vi "Test ConfigurableQMH API.vi"() -> ()   [LabVIEW 2014]
doc: "ConfigurableQMH API Tester."
uses:
  ModuleConfiguration--Cluster.ctl
  ConfigurableQMH.lvlib
panel:
  in  "Active Modules":i32(listbox)
  in  "New Module Name":string
  in  "Modify Configuration":bool
  in  "Configuration":T1
  in  "Run as Singleton?":bool
  in  "Show Block Diagram":bool
  in  "Refresh Modules":bool
  in  "Stop Module":bool
  in  "Run New Module":bool
  in  "Hide Module Panel":bool
  in  "Show Module Panel":bool
  out "Status":string
  # "This VI tests the API for the Module."
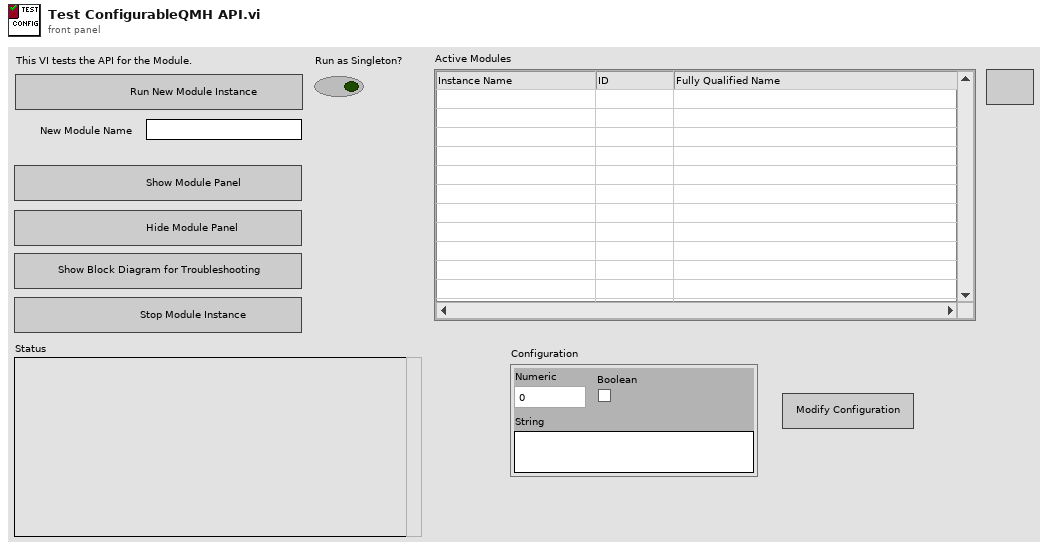
[diagram p1: front panel]
types:
  T1 = typedef "ConfigurableQMH.lvlib/ModuleConfiguration--Cluster.ctl" = cluster{"Numeric":dbl, "Boolean":bool, "String":string}
  T2 = typedef "ConfigurableQMH.lvlib/Broadcast Events--cluster.ctl" = cluster{"Module Did Init":refnum<user-event>, "Status Updated":refnum<user-event>, "Error Reported":refnum<user-event>, "Module Did Stop":refnum<user-event>, "Update Module Execution Status":refnum<user-event>, "Module Configuration":refnum<user-event>}
  T3 = typedef "ConfigurableQMH.lvlib/GetConfiguration (Reply Payload)--cluster.ctl" = cluster{"Configuration":T1, "GetConfiguration_error":errorcluster}
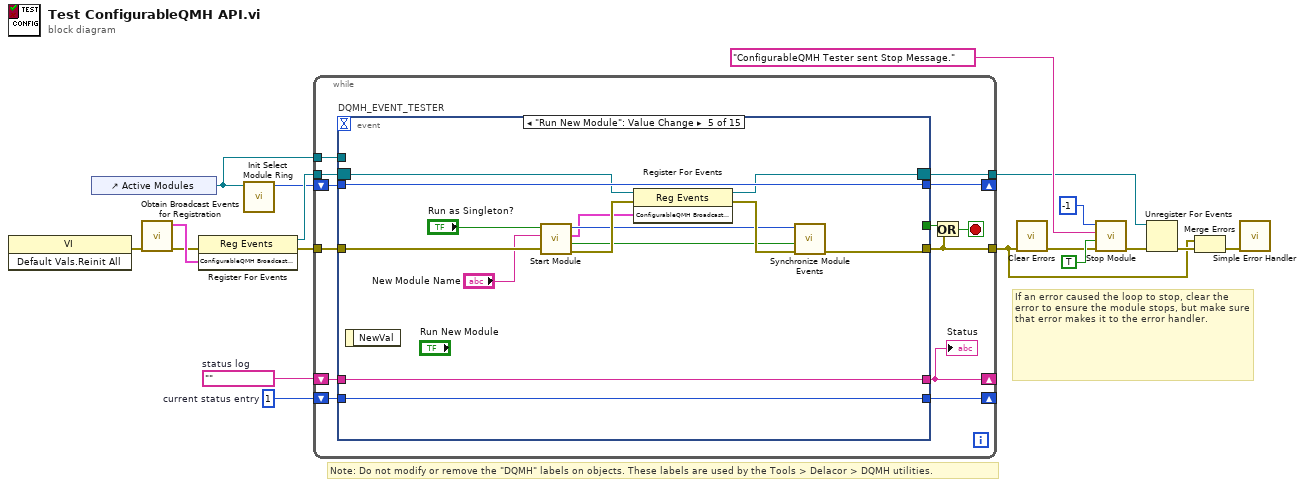
[diagram p0: block diagram]
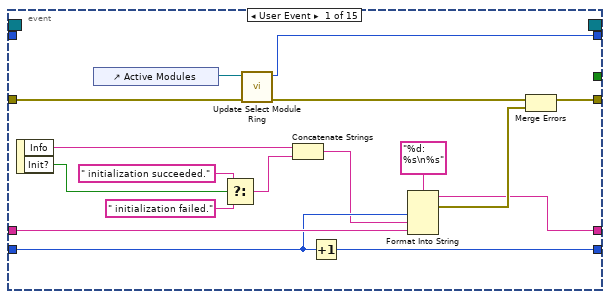
[diagram p2: hidden frame]
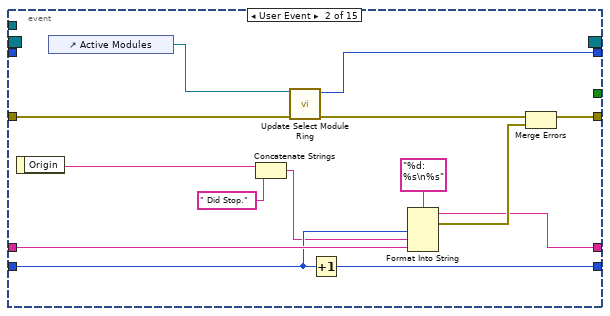
[diagram p3: hidden frame]
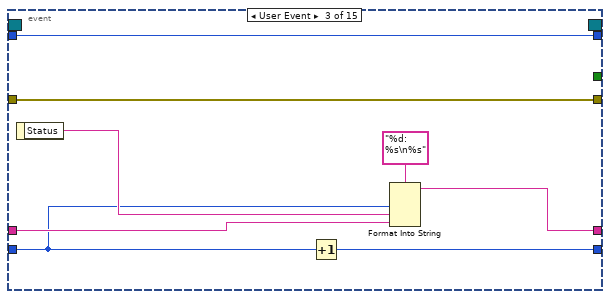
[diagram p4: hidden frame]
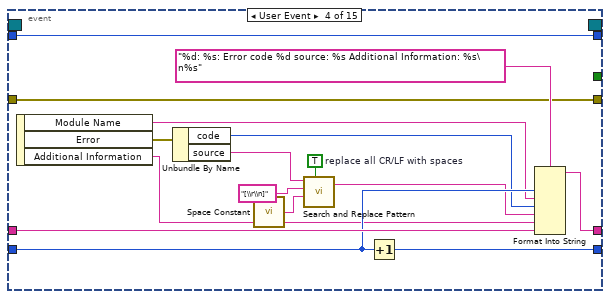
[diagram p5: hidden frame]
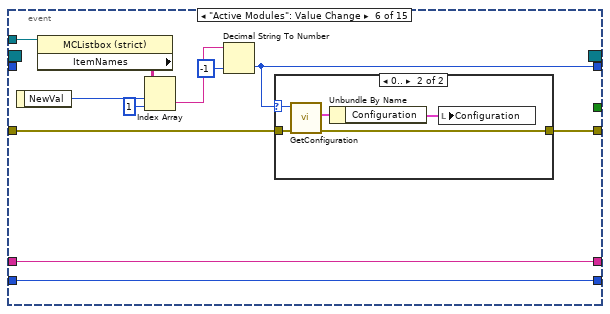
[diagram p6: hidden frame]
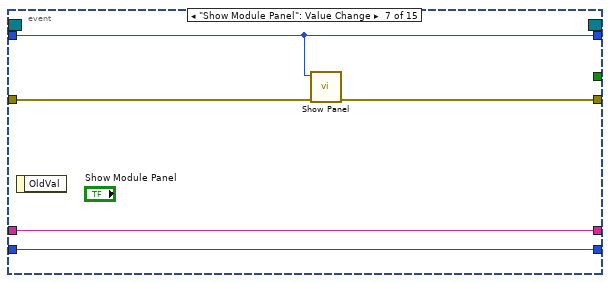
[diagram p8: hidden frame]
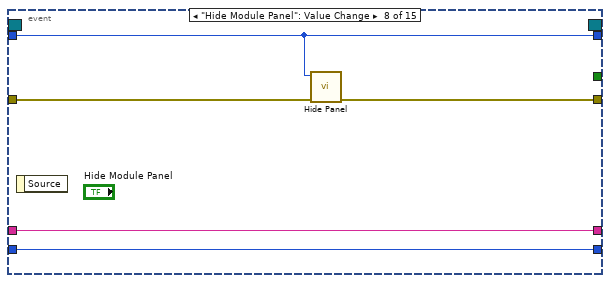
[diagram p9: hidden frame]
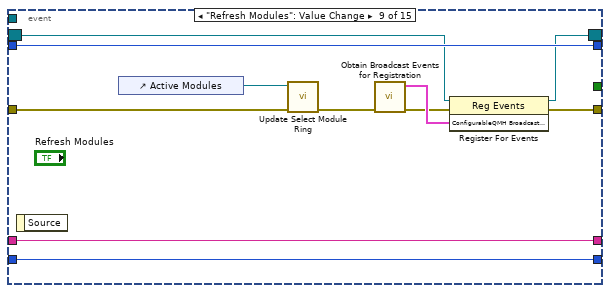
[diagram p10: hidden frame]
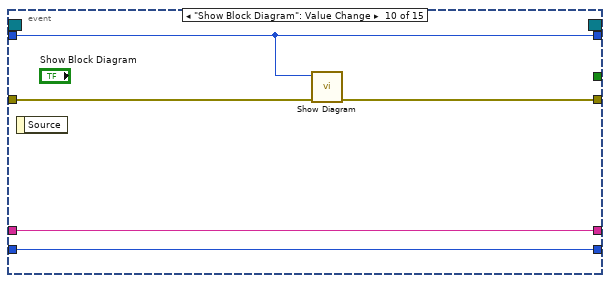
[diagram p11: hidden frame]
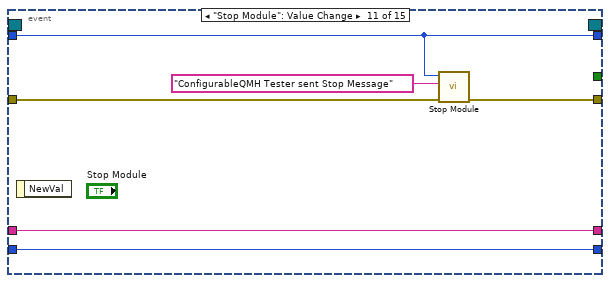
[diagram p12: hidden frame]
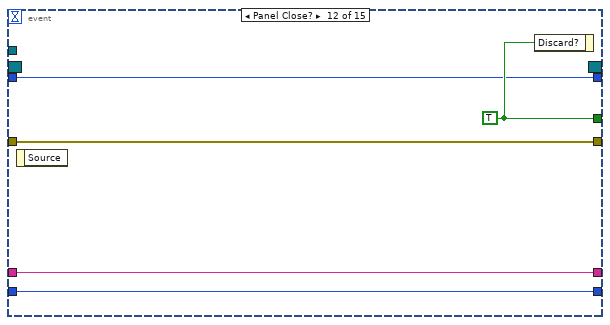
[diagram p13: hidden frame]
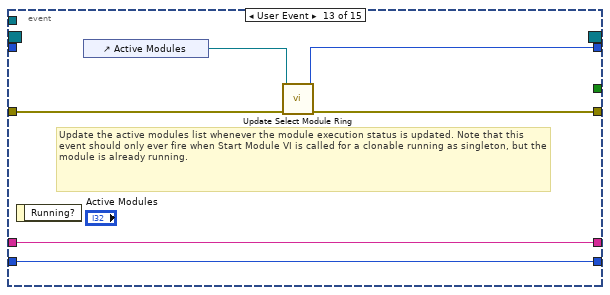
[diagram p14: hidden frame]
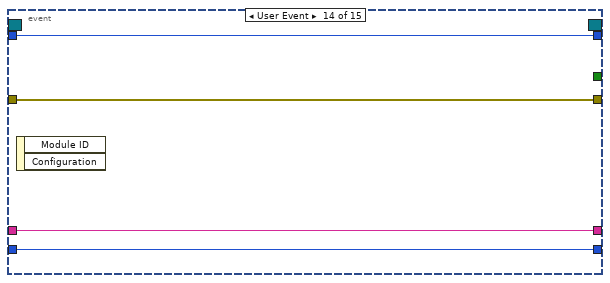
[diagram p15: hidden frame]
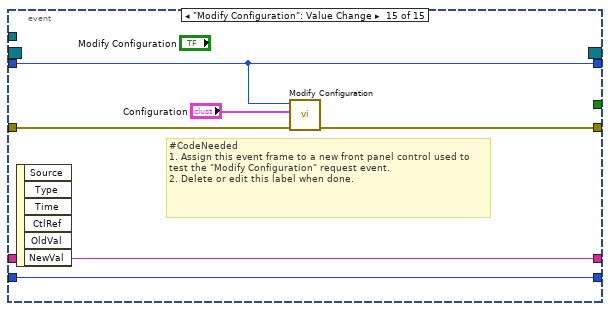
[diagram p16: hidden frame]
diagram:
  w14 = 1  # current status entry
  w15 = ""  # status log
  # "If an error caused the loop to stop, clear the error to ensure the module stops, but make sure that error makes it to the error handler."
  # "Note: Do not modify or remove the \"DQMH\" labels on objects. These labels are used by the Tools > Delacor > DQMH utilities."
  n1 = invoke class="VI" method="Default Vals.Reinit All"() -> (error out=w3:errorcluster)  [unwired: 3 in, 2 out]
  n2 = control-ref of="Active Modules"() -> (w1:refnum<vi>)
  n3 = call "Obtain Broadcast Events for Registration.vi"("error in (no error)"=w3) -> ("error out"=w2:errorcluster, "ConfigurableQMH Broadcast Events"=w12:T2)  [unwired: 9 in]
  n4 = register-events(error in=w2, w12) -> (reference out=w18:refnum<event-registration>, error out=w11:errorcluster)  [unwired: 1 in]
  n5 = call "Init Select Module Ring.vi"("Select Module MCL Ref"=w1) -> ("Value for All Modules"=w13:i32)  [unwired: 8 in, 2 out]
  n6 = while {
    tunnel: w18 -> [w31]
    tunnel: [w20] -> w4
    tunnel: w11 -> [w29]
    shift-right: [w25] -> _
    shift-left: w15 -> [w27]
    shift-right: [w26] -> _
    shift-left: w14 -> [w28]
    shift-right: [w22] -> _
    shift-left: w13 -> [w23]
    tunnel: [w21] -> w8
    tunnel: w1 -> [w19]
    stop <- w24 stop-if-true
    n7 = event "DQMH_EVENT_TESTER" shown="[4] \"Run New Module\": Value Change" {
      selector: w31 -> [_ _ _ _ w94 _ _ _ w134 _ _ _ _ _ _]
      dyn-events: [_ _ _ _ w93 _ _ _ w133 _ _ _ _ _ _] -> w21
      timeout: _ -> [_ _ _ _ _ _ _ _ _ _ _ _ _ _ _]
      tunnel: [_ _ _ _ _ _ _ _ _ _ _ w154 _ _ _] -> w30
      tunnel: [w39 w54 w70 w76 w92 w102 w121 w126 w128 w140 w145 w153 w157 w164 w167] -> w20
      tunnel: w29 -> [w40 w56 w70 w76 w95 w103 w122 w127 w135 w143 w146 w153 w158 w164 w170]
      tunnel: w28 -> [w45 w59 w63 w82 w97 w110 w119 w124 w137 w141 w148 w151 w159 w162 w168]
      tunnel: w27 -> [w46 w60 w66 w84 w98 w111 w120 w125 w138 w142 w149 w152 w160 w163 w169]
      tunnel: [w43 w57 w67 w79 w98 w111 w120 w125 w138 w142 w149 w152 w160 w163 w169] -> w25
      tunnel: [w44 w58 w69 w85 w97 w110 w119 w124 w137 w141 w148 w151 w159 w162 w168] -> w26
      tunnel: w23 -> [_ _ w64 w86 w96 _ w118 w123 w136 w139 w147 w150 _ w161 w166]
      tunnel: [w38 w53 w64 w86 w96 w101 w118 w123 w136 w139 w147 w150 w155 w161 w166] -> w22
      tunnel: w19 -> [_ _ _ _ _ w104 _ _ _ _ _ _ _ _ _]
      event User Event {
        n8 = event-data() -> ("Info"=w42:string, "Init?"=w35:bool)  [unwired: 1 in]
        n9 = control-ref of="Active Modules"() -> (w32:refnum<vi>)
        n10 = Select(t=" initialization succeeded.", s=w35, f=" initialization failed.") -> (s? t:f=w34:string)
        n11 = call "Update Select Module Ring.vi"("error in (no error)"=w40, "Select Module MCL Ref"=w32) -> ("error out"=w33:errorcluster, "New Module Ring Value"=w38:i32)  [unwired: 8 in]
        n12 = Concatenate Strings(w42, w34) -> (w41:string)
        n13 = Increment(x=w45) -> (x+1=w44:i32)
        n14 = Format Into String(format string="%d: %s\n%s", w45, w41, w46) -> (resulting string=w43:string, error out=w48:errorcluster)  [unwired: 2 in]
        n15 = Merge Errors(w33, w48) -> (w39:errorcluster)
      }
      event User Event {
        n16 = event-data() -> ("Origin"=w51:string)  [unwired: 1 in]
        n17 = control-ref of="Active Modules"() -> (w49:refnum<vi>)
        n18 = Concatenate Strings(w51, " Did Stop.") -> (w50:string)
        n19 = call "Update Select Module Ring.vi"("error in (no error)"=w56, "Select Module MCL Ref"=w49) -> ("error out"=w55:errorcluster, "New Module Ring Value"=w53:i32)  [unwired: 8 in]
        n20 = Increment(x=w59) -> (x+1=w58:i32)
        n21 = Format Into String(format string="%d: %s\n%s", w59, w50, w60) -> (resulting string=w57:string, error out=w62:errorcluster)  [unwired: 2 in]
        n22 = Merge Errors(w55, w62) -> (w54:errorcluster)
      }
      event User Event {
        n23 = event-data() -> ("Status"=w65:string)  [unwired: 1 in]
        n24 = Increment(x=w63) -> (x+1=w69:i32)
        n25 = Format Into String(format string="%d: %s\n%s", w63, w65, w66) -> (resulting string=w67:string)  [unwired: 2 in, 1 out]
      }
      event User Event {
        w80 = TRUE  # replace all CR/LF with spaces
        n26 = event-data() -> ("Module Name"=w74:string, "Error"=w73:errorcluster, "Additional Information"=w71:string)  [unwired: 1 in]
        n27 = Unbundle By Name(w73) -> ("code"=w75:i32, "source"=w77:string)
        n28 = call <vilib>:"Space Constant.vi"() -> ("String"=w81:string)
        n29 = call <vilib>:"Search and Replace Pattern.vi"("string"=w77, "regular expression (\"\")"="[\\r\\n]" ("regular expression (\"\")"), "replace string (\"\")"=w81, "replace all? (F)"=w80) -> ("result string"=w78:string)  [unwired: 1 in, 1 out]
        n30 = Increment(x=w82) -> (x+1=w85:i32)
        n31 = Format Into String(format string="%d: %s: Error code %d source: %s Additional Information: %s\n%s", w82, w74, w75, w78, w71, w84) -> (resulting string=w79:string)  [unwired: 2 in, 1 out]
      }
      event "Run New Module": Value Change {
        n32 = event-data() -> ()  [unwired: 1 in, 1 out]
        n33 = call "Start Module.vi"("error in (no error)"=w95, "Module Name (empty: default)"="New Module Name", "Run as Singleton? (F)"="Run as Singleton?") -> ("error out"=w99:errorcluster, "Wait for Event Sync?"=w90:bool, "ConfigurableQMH Broadcast Events"=w89:T2, "Module ID"=w91:i32)  [unwired: 5 in]
        n34 = register-events(reference=w94, error in=w99, w89) -> (reference out=w93:refnum<event-registration>, error out=w100:errorcluster)
        n35 = call "Synchronize Module Events.vi"("error in (no error)"=w100, "Wait for Event Sync?"=w90, "Module ID"=w91) -> ("error out"=w92:errorcluster)  [unwired: 7 in, 1 out]
      }
      event "Active Modules": Value Change {
        n36 = event-data() -> ("NewVal"=w108:i32)  [unwired: 1 in]
        n37 = property class="MCListbox (strict)"(reference=w104) -> ("ItemNames"=w109:string[][])  [unwired: 1 in, 2 out]
        n38 = Index Array(array=w109, index (row)=w108, index (col)=1 ("disabled index (col)")) -> (element=w106:string)
        n39 = Decimal String To Number(string=w106, default (0L)=-1 ("default (0 I32)")) -> (number=w101:i32)  [unwired: 1 in, 1 out]
        n40 = case shown="0.." w101 {
          selector: w101 -> [_ w113]
          tunnel: w103 -> [w112 w115]
          tunnel: [w112 w114] -> w102
          frame Default {
          }
          frame 0.. {
            n41 = call "GetConfiguration.vi"("error in (no error)"=w115, "Module ID"=w113) -> ("error out"=w114:errorcluster, "Reply Payload"=w117:T3)  [unwired: 7 in, 1 out]
            n42 = Unbundle By Name(w117) -> ("Configuration"=w116:T1)
            n43 = local write "Configuration"(w116) -> ()
          }
        }
      }
      event "Show Module Panel": Value Change {
        n44 = event-data() -> ()  [unwired: 1 in, 1 out]
        n45 = call "Show Panel.vi"("error in (no error)"=w122, "Module ID"=w118) -> ("error out"=w121:errorcluster)  [unwired: 9 in]
      }
      event "Hide Module Panel": Value Change {
        n46 = event-data() -> ()  [unwired: 1 in, 1 out]
        n47 = call "Hide Panel.vi"("error in (no error)"=w127, "Module ID"=w123) -> ("error out"=w126:errorcluster)  [unwired: 9 in]
      }
      event "Refresh Modules": Value Change {
        n48 = event-data() -> ()  [unwired: 1 in, 1 out]
        n49 = control-ref of="Active Modules"() -> (w130:refnum<vi>)
        n50 = call "Update Select Module Ring.vi"("error in (no error)"=w135, "Select Module MCL Ref"=w130) -> ("error out"=w131:errorcluster)  [unwired: 8 in, 1 out]
        n51 = call "Obtain Broadcast Events for Registration.vi"("error in (no error)"=w131) -> ("error out"=w129:errorcluster, "ConfigurableQMH Broadcast Events"=w132:T2)  [unwired: 9 in]
        n52 = register-events(reference=w134, error in=w129, w132) -> (reference out=w133:refnum<event-registration>, error out=w128:errorcluster)
      }
      event "Show Block Diagram": Value Change {
        n53 = event-data() -> ()  [unwired: 1 in, 1 out]
        n54 = call "Show Diagram.vi"("error in (no error)"=w143, "Module ID"=w139) -> ("error out"=w140:errorcluster)  [unwired: 9 in]
      }
      event "Stop Module": Value Change {
        n55 = event-data() -> ()  [unwired: 1 in, 1 out]
        n56 = call "Stop Module.vi"("error in (no error)"=w146, "Origin"="ConfigurableQMH Tester sent Stop Message", "Module ID"=w147) -> ("error out"=w145:errorcluster)  [unwired: 8 in]
      }
      event Panel Close? {
        w154 = TRUE ("Discard?")
        n57 = event-data() -> ()  [unwired: 1 in, 1 out]
        n58 = event-data("Discard?"=w154) -> ()  [unwired: 1 in, 1 out]
      }
      event User Event {
        # "Update the active modules list whenever the module execution status is updated. Note that this event should only ever fire when Start Module VI is called for a clonable running as singleton, but the module is already running."
        n59 = event-data() -> ()  [unwired: 1 in, 1 out]
        n60 = control-ref of="Active Modules"() -> (w156:refnum<vi>)
        n61 = call "Update Select Module Ring.vi"("error in (no error)"=w158, "Select Module MCL Ref"=w156) -> ("error out"=w157:errorcluster, "New Module Ring Value"=w155:i32)  [unwired: 8 in]
      }
      event User Event {
        n62 = event-data() -> ()  [unwired: 1 in, 2 out]
      }
      event "Modify Configuration": Value Change {
        # "#CodeNeeded\n1. Assign this event frame to a new front panel control used to test the \"Modify Configuration\" request event.\n2. Delete or edit this label when done."
        n63 = event-data() -> ()  [unwired: 1 in, 6 out]
        n64 = call "Modify Configuration.vi"("error in (no error)"=w170, "Configuration"="Configuration", "Module ID"=w166) -> ("error out"=w167:errorcluster)  [unwired: 8 in]
      }
    }
    "Status" <- w25
    n65 = Or(x=w30, y=w20) -> (x .or. y?=w24:bool)
  }
  n66 = call <vilib>:"Clear Errors.vi"("error in (no error)"=w4) -> ("error out"=w6:errorcluster)  [unwired: 5 in, 1 out]
  n67 = call "Stop Module.vi"("error in (no error)"=w6, "Wait for Module to stop? (F)"=TRUE ("Wait for Module to stop?"), "Origin"="ConfigurableQMH Tester sent Stop Message.", "Module ID"=-1 ("Stop all")) -> ("error out"=w16:errorcluster)  [unwired: 7 in]
  n68 = Unregister For Events(event registration refnum=w8, error in=w16) -> (error out=w17:errorcluster)
  n69 = Merge Errors(w4, w17) -> (w5:errorcluster)
  n70 = call <vilib>:"Simple Error Handler.vi"("error in (no error)"=w5) -> ()  [unwired: 4 in, 5 out]
